vi "Read Data.vi"(8 "error in (no error)":errorcluster, 11 "String Request Message in":refnum<class "String Request Message.lvclass">) -> (0 "error out":errorcluster, 2 "Data":string, 3 "String Request Message out":refnum<class "String Request Message.lvclass">)   [LabVIEW 2017, in "String Request Message.lvclass"]
uses:
  String Request Message.lvclass
  String Request Message.lvclass/String Request Message.ctl
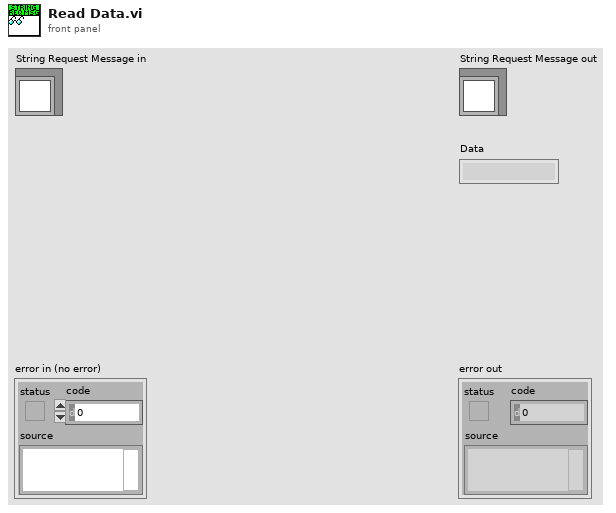
[diagram p1: front panel]
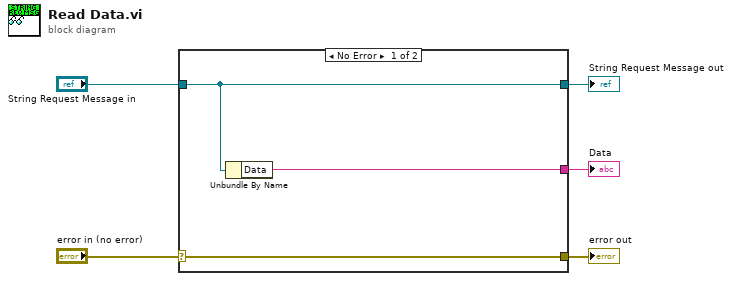
[diagram p0: block diagram]
diagram:
  n1 = case shown="No Error" "error in (no error)" {
    selector: "error in (no error)" -> [w8 w9]
    tunnel: [w8 w9] -> w4
    tunnel: [w7 w10] -> w2
    tunnel: "String Request Message in" -> [w7 w10]
    tunnel: [w6 _] -> w1
    frame No Error {
      n2 = Unbundle By Name(w7) -> ("Data"=w6:string)
    }
    frame Error {
    }
  }
  "error out" <- w4
  "String Request Message out" <- w2
  "Data" <- w1
